vi "open-image.vi"() -> ()   [LabVIEW 2021]
uses:
  open-image-states.ctl
  <vilib>/Utility/file.llb/Read Delimited Spreadsheet (DBL).vi
panel:
  in  "row index":i32
  out "Graph":dbl[](graph)
  out "Graph 2":dbl[](graph)
  in  "column index":i32
  in  "Close":bool
  in  "Open":bool
  in  "Interpolation Method":i32(ring) items=["nearest", "bilinear", "bicubic", "bicubic spline"]
  in  "N Times Interpolation":i32=20
  in  "Open File (.csv)":path caption="Path"
  out "Intensity Graph of The Original Data":dbl[][](graph)
  in  "Save as .png":bool
  in  "Intensity Scale Values-Colors":cluster{"Value":dbl, "Color":u32}[](array[cluster])=[{"Value"=0.0, "Color"=0}, {"Value"=0.5, "Color"=16716306}, {"Value"=1.0, "Color"=16187225}]
  out "Intensity Graph of The Interpolated Data":dbl[][](graph)
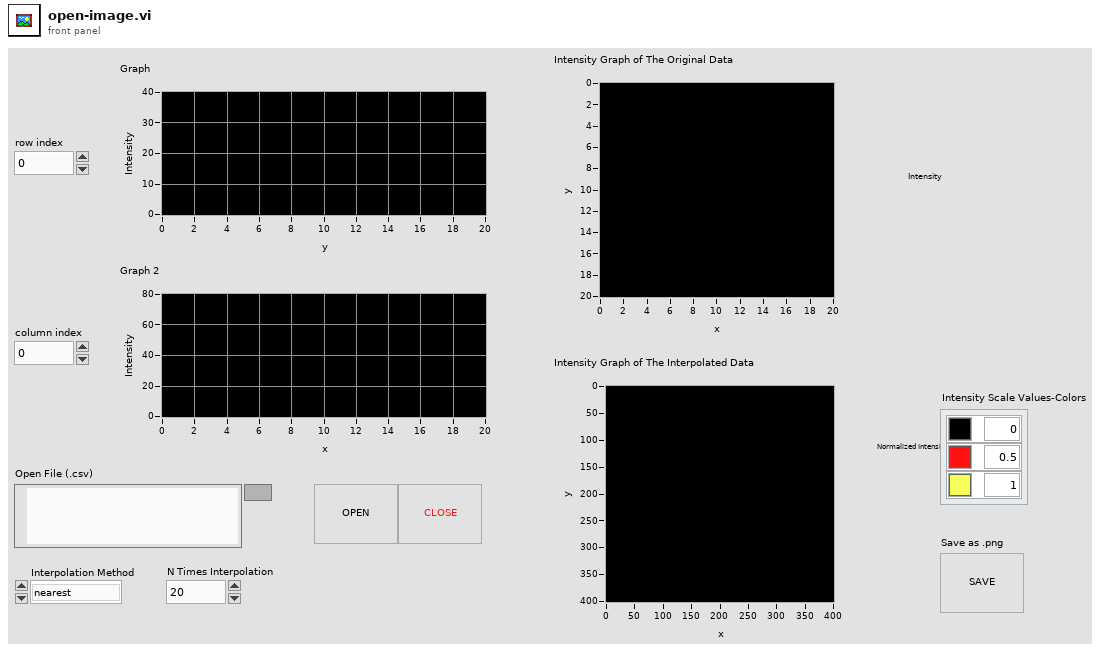
[diagram p1: front panel]
types:
  T1 = typedef "open-image-states.ctl" = enum16{"init", "idle", "open", "exit", "error", "save"}
  T2 = typedef "imagedata.ctl" = cluster{"image type":i32, "image depth":i32, "image":u8[], "mask":u8[], "colors":u32[], "Rectangle":cluster{"left":i16, "top":i16, "right":i16, "bottom":i16}}
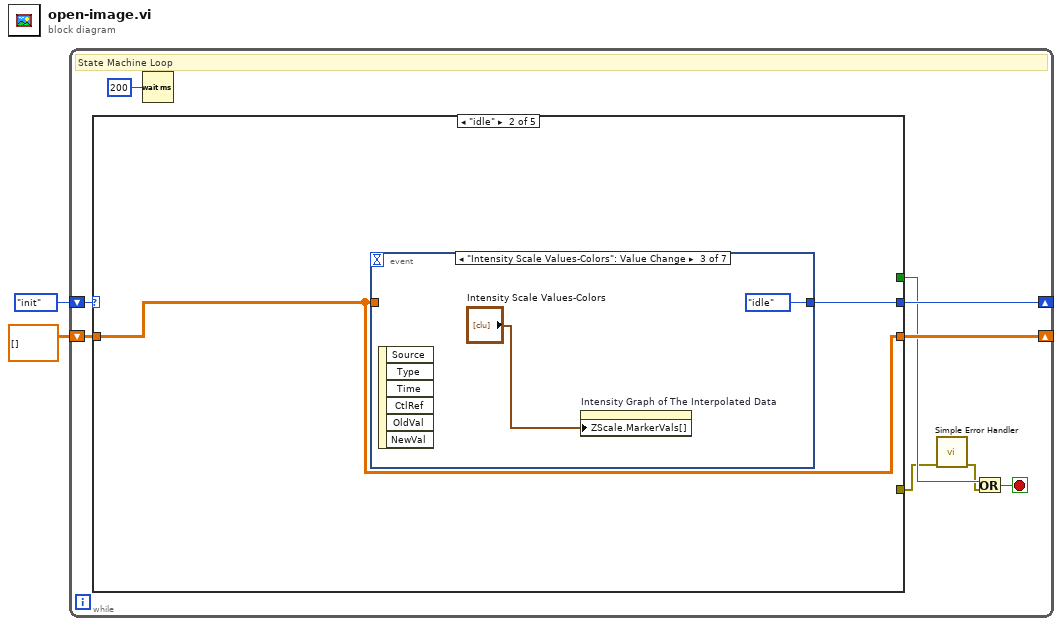
[diagram p0: block diagram]
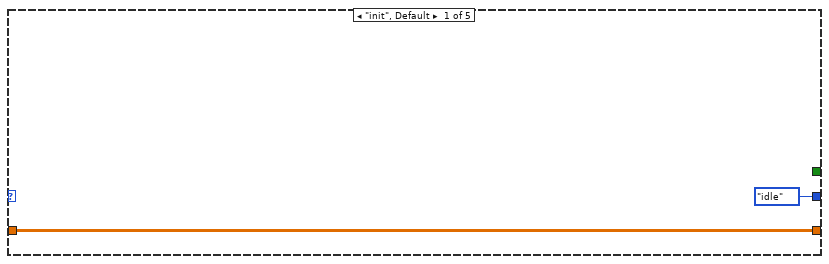
[diagram p2: hidden frame]
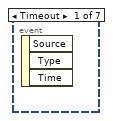
[diagram p3: hidden frame]
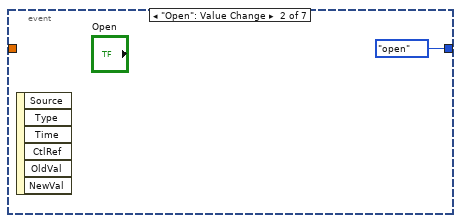
[diagram p4: hidden frame]
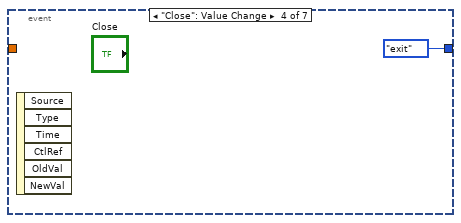
[diagram p5: hidden frame]
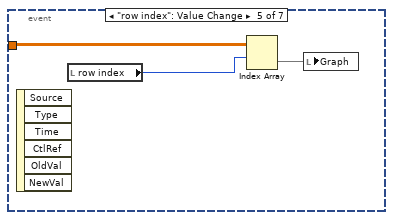
[diagram p6: hidden frame]
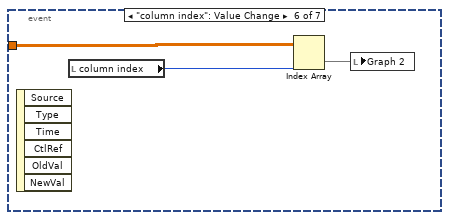
[diagram p7: hidden frame]
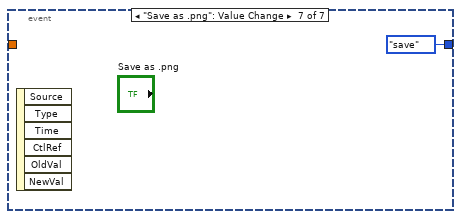
[diagram p8: hidden frame]
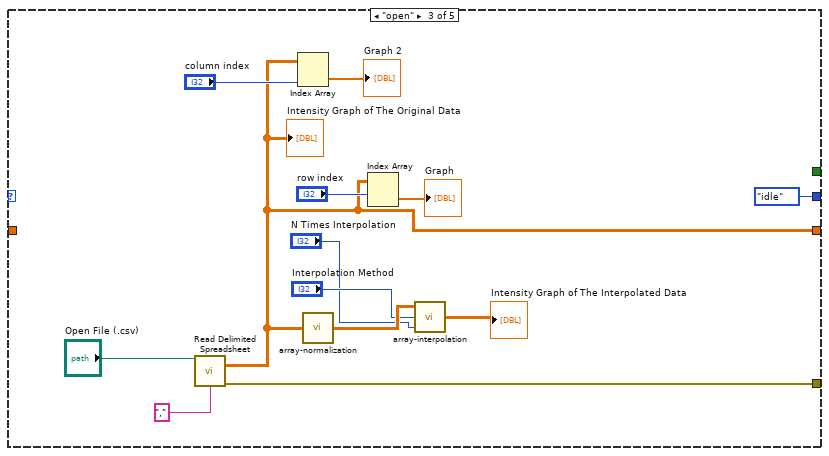
[diagram p9: hidden frame]
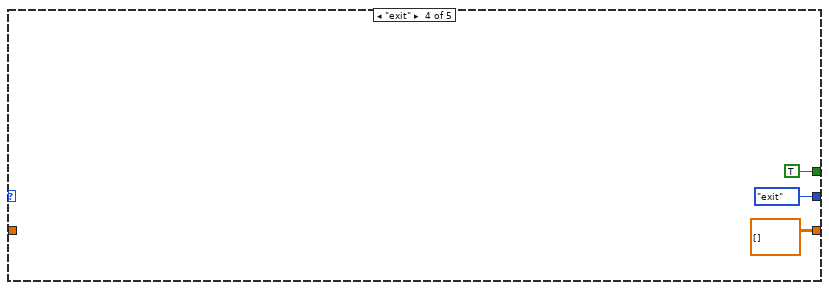
[diagram p10: hidden frame]
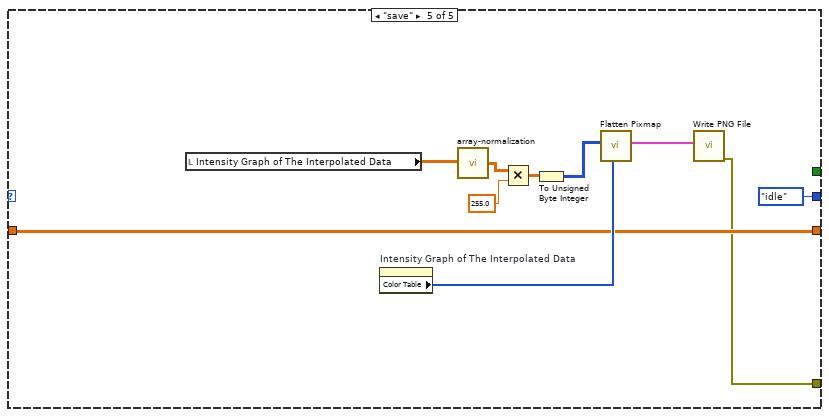
[diagram p11: hidden frame]
diagram:
  n1 = while {
    shift-right: [w8] -> _
    shift-left: dbl[][] [] -> [w7]
    shift-right: [w9] -> _
    shift-left: open-image-states."init" -> [w10]
    stop <- w5 stop-if-true
    # "State Machine Loop"
    n2 = case shown="\"idle\"" w10 {
      tunnel: [open-image-states."idle" w15 open-image-states."idle" open-image-states."exit" open-image-states."idle"] -> w9
      tunnel: [w12 w14 w32 dbl[][] [] ("all rows") w45] -> w8
      tunnel: w7 -> [w12 w14 _ _ w45]
      tunnel: [_ _ _ TRUE _] -> w6
      tunnel: [_ _ w27 _ w43] -> w4
      frame "init", Default {
      }
      frame "idle" {
        n3 = event shown="[2] \"Intensity Scale Values-Colors\": Value Change" {
          selector: _ -> [_ _ _ _ _ _ _]
          dyn-events: _ -> [_ _ _ _ _ _ _]
          timeout: _ -> [_ _ _ _ _ _ _]
          tunnel: [_ open-image-states."open" open-image-states."idle" open-image-states."exit" _ _ open-image-states."save"] -> w15
          tunnel: w14 -> [_ _ _ _ w22 w25 _]
          event Timeout {
            n4 = event-data() -> ()  [unwired: 1 in, 3 out]
          }
          event "Open": Value Change {
            n5 = event-data() -> ()  [unwired: 1 in, 6 out]
          }
          event "Intensity Scale Values-Colors": Value Change {
            n6 = event-data() -> ()  [unwired: 1 in, 6 out]
            n7 = property on="Intensity Graph of The Interpolated Data" class="IntGraph (strict)"("ZScale.MarkerVals[]"="Intensity Scale Values-Colors") -> ()  [unwired: 2 in, 2 out]
          }
          event "Close": Value Change {
            n8 = event-data() -> ()  [unwired: 1 in, 6 out]
          }
          event "row index": Value Change {
            n9 = event-data() -> ()  [unwired: 1 in, 6 out]
            n10 = local read "row index"() -> (w20:i32)
            n11 = Index Array(array=w22, index (row)=w20) -> (element=w21:dbl[])  [unwired: 1 in]
            n12 = local write "Graph"(w21) -> ()
          }
          event "column index": Value Change {
            n13 = event-data() -> ()  [unwired: 1 in, 6 out]
            n14 = local read "column index"() -> (w23:i32)
            n15 = Index Array(array=w25, index (col)=w23) -> (element=w24:dbl[])  [unwired: 1 in]
            n16 = local write "Graph 2"(w24) -> ()
          }
          event "Save as .png": Value Change {
            n17 = event-data() -> ()  [unwired: 1 in, 6 out]
          }
        }
      }
      frame "open" {
        n18 = call-poly <vilib>:"Read Delimited Spreadsheet.vi"("file path (dialog if empty)"="Open File (.csv)", "delimiter (\\t)"="," ("delimiter (\\t)")) -> ("all rows"=w32:dbl[][], "error out"=w27:errorcluster)  [unwired: 8 in, 4 out]
        "Intensity Graph of The Original Data" <- w32
        n19 = Index Array(array=w32, index (col)="column index") -> (element=→"Graph 2":dbl[])  [unwired: 1 in]
        n20 = call "array-normalization.vi"("Array"=w32) -> ("x/y"=w30:dbl[][])
        n21 = Index Array(array=w32, index (row)="row index") -> (element=→"Graph":dbl[])  [unwired: 1 in]
        n22 = call "array-interpolation.vi"("N Times Interpolation"="N Times Interpolation", "Interpolation Method"="Interpolation Method", "2D Data"=w30) -> ("Interpolated Data"=→"Intensity Graph of The Interpolated Data":dbl[][])
      }
      frame "exit" {
      }
      frame "save" {
        n23 = local read "Intensity Graph of The Interpolated Data"() -> (w52:dbl[][])
        n24 = property on="Intensity Graph of The Interpolated Data" class="IntGraph (strict)"() -> ("Color Table"=w47:u32[])  [unwired: 2 in, 2 out]
        n25 = call "array-normalization.vi"("Array"=w52) -> ("x/y"=w50:dbl[][])
        n26 = Multiply(x=w50, y=255.0) -> (x*y=w49:dbl[][])
        n27 = To Unsigned Byte Integer(number=w49) -> (unsigned 8bit integer=w48:u8[][])
        n28 = call <vilib>:"Flatten Pixmap.vi"("colors"=w47, "8-bit pixmap"=w48) -> ("image data"=w46:T2)  [unwired: 9 in]
        n29 = call <vilib>:"Write PNG File.vi"("image data"=w46) -> ("error out"=w43:errorcluster)  [unwired: 9 in, 1 out]
      }
    }
    n30 = Wait (ms)(milliseconds to wait=u32 200) -> ()  [unwired: 1 out]
    n31 = call <vilib>:"Simple Error Handler.vi"("error in (no error)"=w4) -> ("error out"=w3:errorcluster)  [unwired: 4 in, 4 out]
    n32 = Or(x=w6, y=w3) -> (x .or. y?=w5:bool)
  }
